vi "control output.vi"(10 "DACB":dbl step=0.1 format="%.4f", 11 "DACA":dbl step=0.1 format="%.4f") -> ()   [LabVIEW 2015]
panel:
  in  "FirstFound":bool=TRUE
  in  "Address":string="1"
  out "Error Message":string
  out "error out":errorcluster
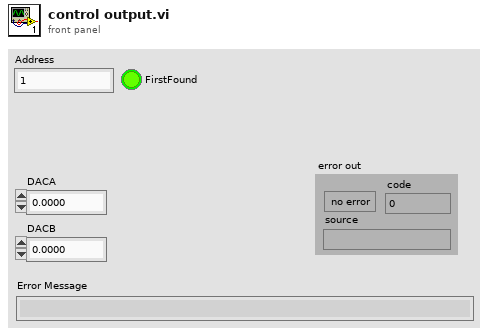
[diagram p1: front panel]
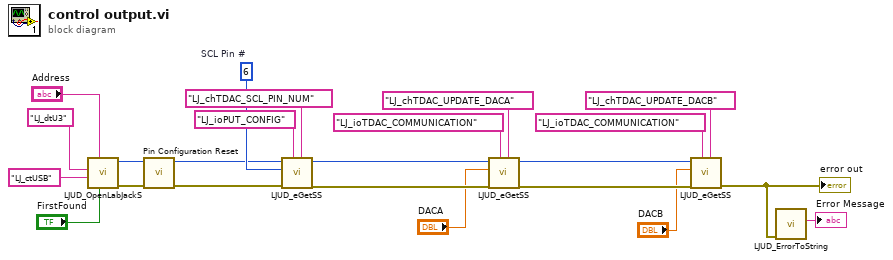
[diagram p0: block diagram]
diagram:
  w14 = 6  # SCL Pin #
  n1 = call "LJUD_OpenLabJackS.vi"("FirstFound"="FirstFound", "Address"="Address", "ConnectionType"="LJ_ctUSB", "DeviceType"="LJ_dtU3") -> ("error out"=w17:errorcluster, "Handle"=w18:i32)  [unwired: 5 in, 1 out]
  n2 = call "Pin Configuration Reset.vi"("error in"=w17, "Handle In"=w18) -> ("error out"=w12:errorcluster, "Handle Out"=w13:i32)  [unwired: 8 in]
  n3 = call "LJUD_eGetSS.vi"("Channel"="LJ_chTDAC_SCL_PIN_NUM", "IOType"="LJ_ioPUT_CONFIG", "error in"=w12, "Value Write"=w14, "Handle In"=w13) -> ("error out"=w8:errorcluster, "Handle Out"=w9:i32)  [unwired: 4 in, 1 out]
  n4 = call "LJUD_eGetSS.vi"("Channel"="LJ_chTDAC_UPDATE_DACA", "IOType"="LJ_ioTDAC_COMMUNICATION", "error in"=w8, "Value Write"="DACA", "Handle In"=w9) -> ("error out"=w3:errorcluster, "Handle Out"=w4:i32)  [unwired: 4 in, 1 out]
  n5 = call "LJUD_eGetSS.vi"("Channel"="LJ_chTDAC_UPDATE_DACB", "IOType"="LJ_ioTDAC_COMMUNICATION", "error in"=w3, "Value Write"="DACB", "Handle In"=w4) -> ("error out"=w2:errorcluster)  [unwired: 4 in, 2 out]
  "error out" <- w2
  n6 = call "LJUD_ErrorToString.vi"("error in"=w2) -> ("String"=→"Error Message":string)  [unwired: 10 in]
